vi "Receiver_Monokrom_Fix.vi"() -> ()   [LabVIEW 2018]
panel:
  in  "Python version":string="3.12.3"
  in  "Python Path Decoder Huffman":path=path "D:/PAKPRI_LAST/PAKPRI/huffman_decoder.py"
  out "Numeric":i32
  out "SNR":dbl
  out "Constellation Diagram Receiver":cdb[](graph)
  out "0, 2":i16[][](array[numeric])
  in  "Image File Reference":path=path "D:/Thesis Pak Pri/boo.bmp"
  out "x/y 3":dbl
  out "BER":dbl
  out "Output Image":picture
  in  "Width":i32=256
  in  "Height":i32=256
  out "Preamble Detected?":bool
  in  "Bit length (set)":i32=3600
  out "sisa bagi":i32
  out "hasil bagi":i32
  out "iterasi":i32
  in  "Modulation parameter":T1
  out "created new?":bool
  out "SIG valid?":bool
  in  "stop":bool
  out "USRP CoercedParamters":T2={"coerced IQ rate"=100000.0, "coerced carrier frequency"=100000.0, "coerced gain"=0.0} {"coerced gain" format="%#_6f"; "coerced carrier frequency" format="%#_6p"; "coerced IQ rate" format="%#_6p"}
  out "error out":errorcluster
  in  "Trigger level":dbl=0.005 format="%f"
  in  "error in (no error)":errorcluster
  in  "USRP ControledParameters":T3={"active antenna"="RX1", "gain"=0.0, "carrier frequency"=915000000.0, "IQ rate"=1000000.0} {"IQ rate" format="%#_6p"; "carrier frequency" format="%#_6p"; "gain" format="%#_6f"}
  in  "device names":refnum<k15>="192.168.10.4"
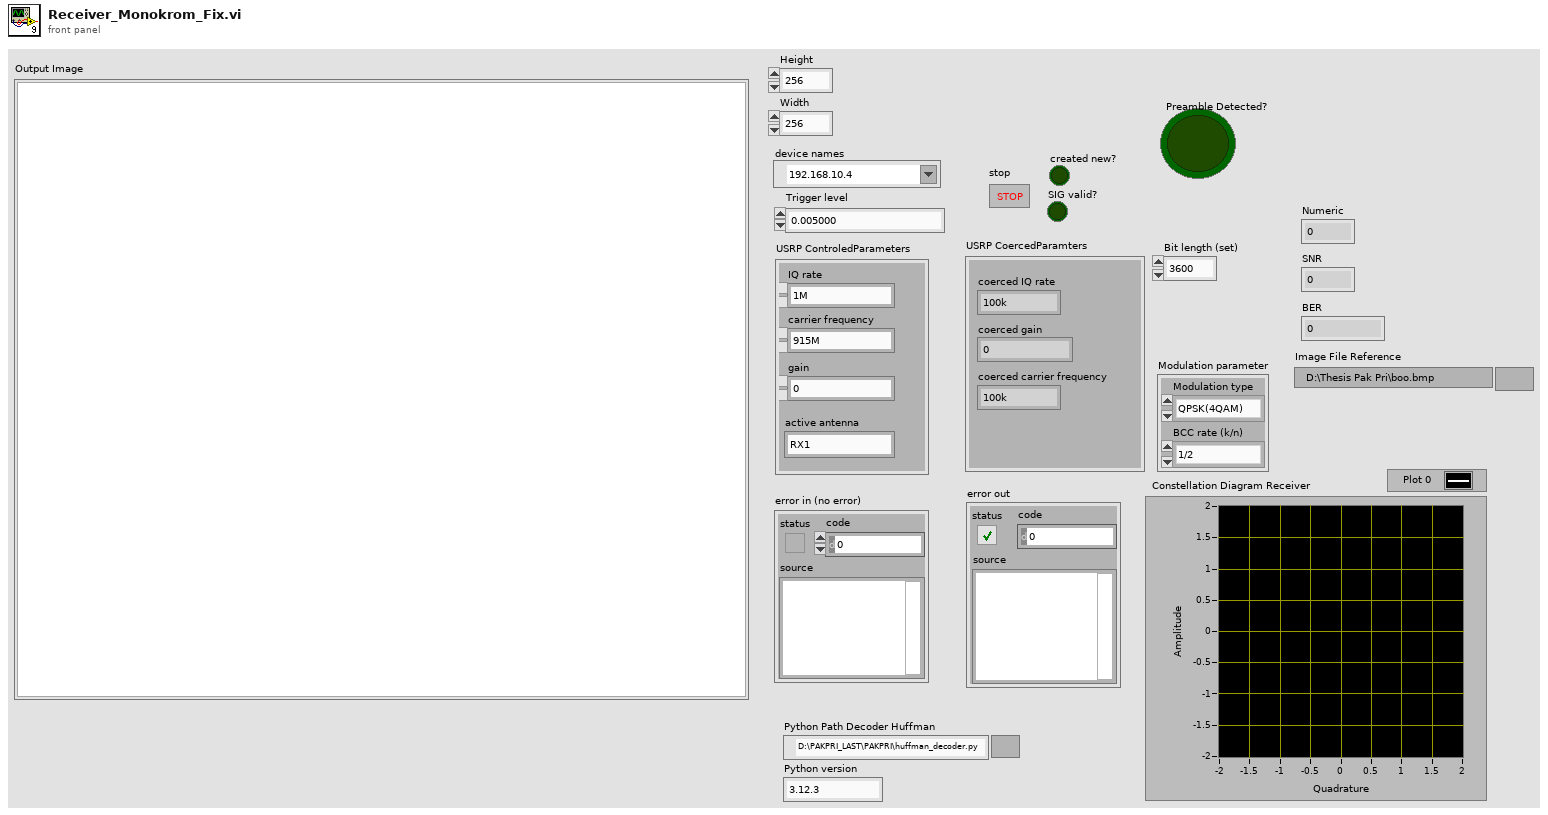
[diagram p1: front panel]
types:
  T1 = cluster{"Modulation type":enum16{"QPSK(4QAM)", "64QAM", "16QAM", "BPSK"}, "BCC rate (k/n)":enum16{"1/2", "2/3", "3/4"}}
  T2 = cluster{"coerced IQ rate":dbl, "coerced carrier frequency":dbl, "coerced gain":dbl}
  T3 = cluster{"active antenna":string, "gain":dbl, "carrier frequency":dbl, "IQ rate":dbl}
  T4 = typedef "imagedata.ctl" = cluster{"image type":i32, "image depth":i32, "image":u8[], "mask":u8[], "colors":u32[], "Rectangle":cluster{"left":i16, "top":i16, "right":i16, "bottom":i16}}
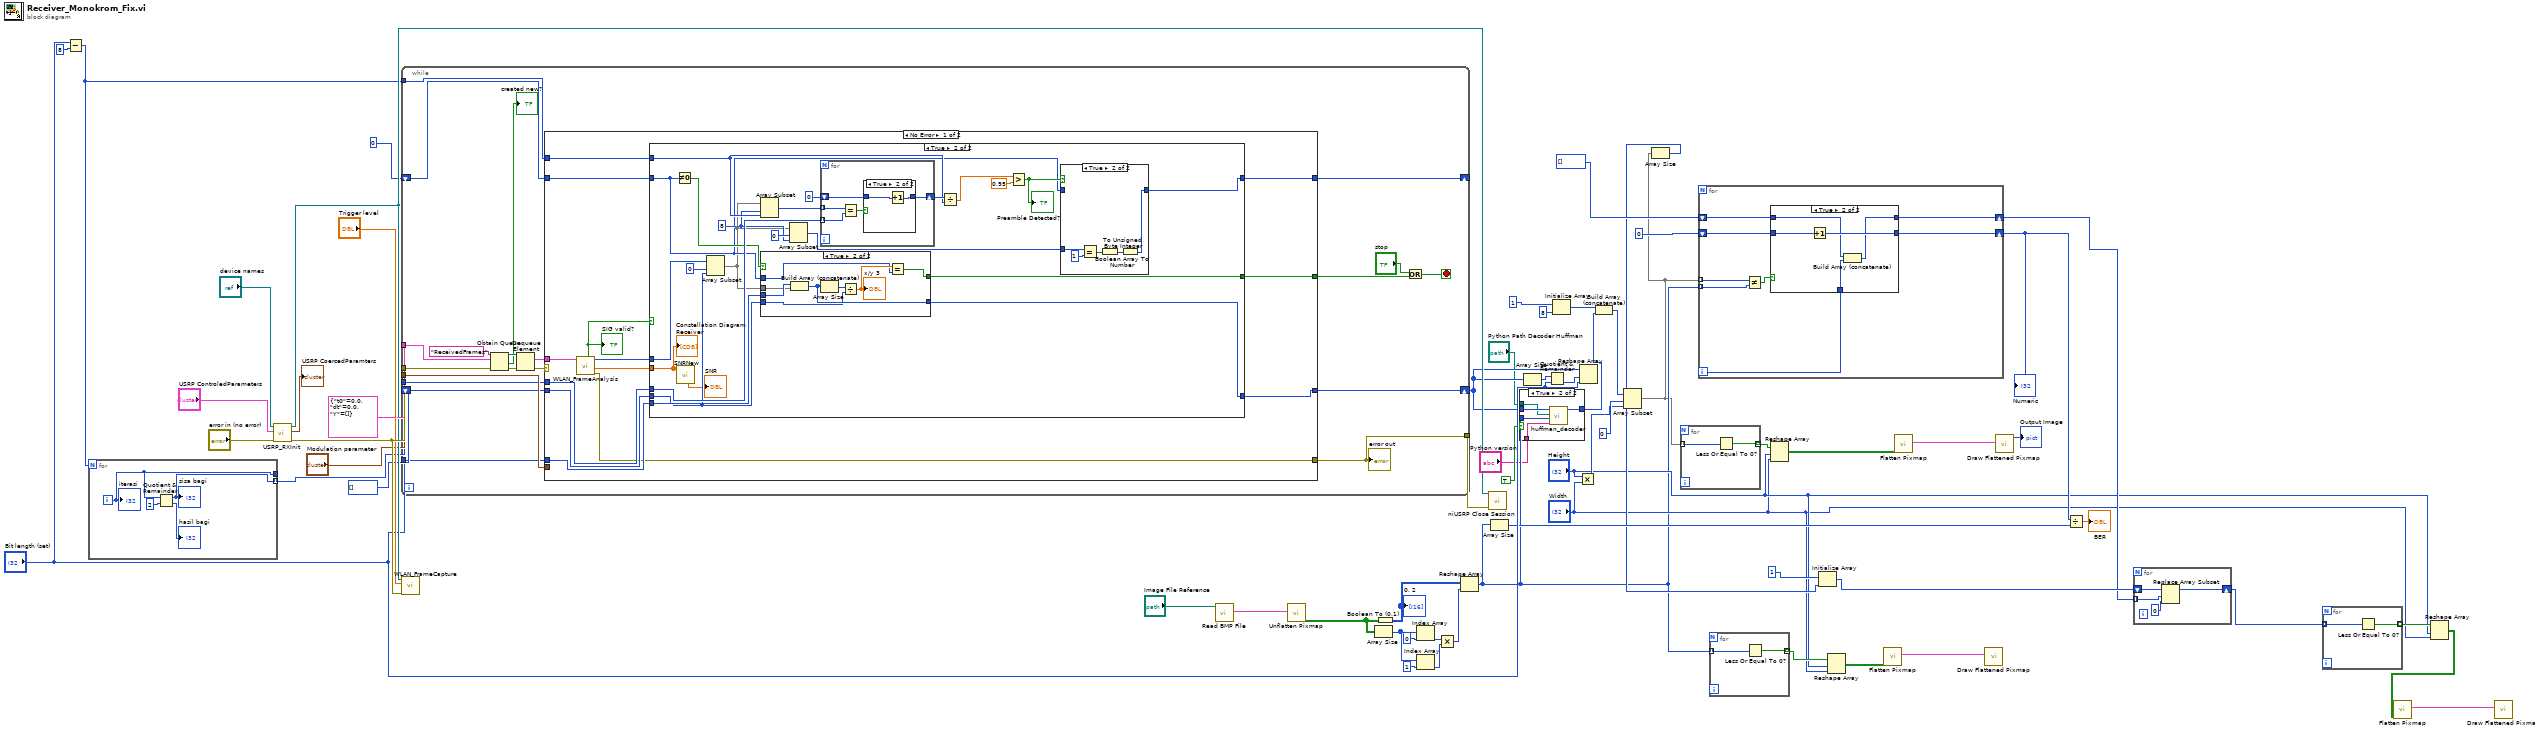
[diagram p0: block diagram]
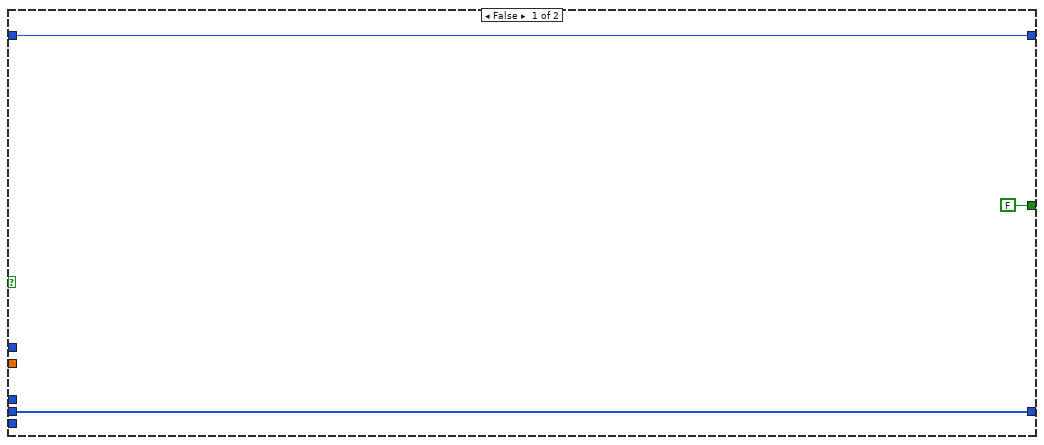
[diagram p4: hidden frame]
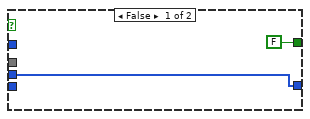
[diagram p5: hidden frame]
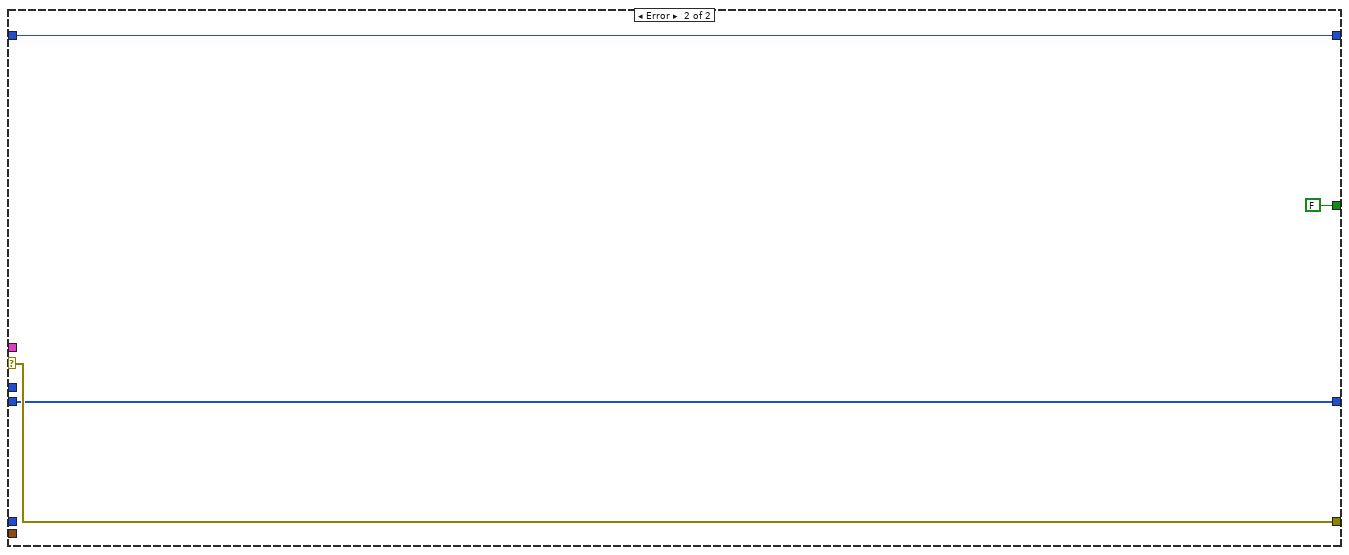
[diagram p8: hidden frame]
diagram:
  n1 = Subtract(x="Bit length (set)", y=8) -> (x-y=w52:i32)
  n2 = for {
    N: w52 -> [_]
    tunnel: [w65] -> _
    tunnel: [w64] -> w51 mode=indexing
    i -> [w65]
    n3 = Quotient & Remainder(x=w65, y=2) -> (x-y*floor(x/y)=w64:i32, floor(x/y)=→"hasil bagi":i32)
    "sisa bagi" <- w64
    "iterasi" <- w65
  }
  n4 = call "USRP_RXInit.vi"("device names"="device names", "USRP ControledParameters"="USRP ControledParameters", "error in (no error)"="error in (no error)") -> ("session handle out"=w55:refnum<k15>, "USRP CoercedParamters"=→"USRP CoercedParamters":T2, "error out"=w59:errorcluster)  [unwired: 5 in]
  n5 = while {
    tunnel: w59 -> [w86]
    tunnel: cluster{"t0":dbl, "dt":dbl, "Y":cdb[]} {"t0"=0.0, "dt"=0.0, "Y"=[]} ("data") -> [w87]
    tunnel: [w79] -> w56
    tunnel: "Modulation parameter" -> [w78]
    tunnel: "Bit length (set)" -> [w77]
    tunnel: w52 -> [w76]
    tunnel: w51 -> [w75]
    shift-right: [w73] -> _
    shift-left: 0 -> [w74]
    shift-right: [w71] -> w25
    shift-left: i32[] [] -> [w72]
    stop <- w68 stop-if-true
    n6 = Obtain Queue(name (unnamed)="ReceivedFrames", element data type=w87, error in (no error)=w86) -> (queue out=w85:refnum<queue>, created new?=→"created new?":bool, error out=w82:errorcluster)  [unwired: 2 in]
    n7 = Dequeue Element(queue=w85, error in (no error)=w82) -> (element=w83:cluster{"t0":dbl, "dt":dbl, "Y":cdb[]}, error out=w84:errorcluster)  [unwired: 1 in, 2 out]
    n8 = case shown="No Error" w84 {
      selector: w84 -> [_ w154]
      tunnel: w83 -> [w92 _]
      tunnel: [w91 w154] -> w79
      tunnel: w78 -> [_ _]
      tunnel: w77 -> [w100 _]
      tunnel: w76 -> [w99 _]
      tunnel: w75 -> [w98 _]
      tunnel: w74 -> [w97 w153]
      tunnel: [w96 w153] -> w73
      tunnel: w72 -> [w95 w152]
      tunnel: [w94 w152] -> w71
      tunnel: [w93 FALSE] -> w69
      frame No Error {
        n9 = call "WLAN_FrameAnalysis.vi"("input cluster"=w92) -> ("error out"=w91:errorcluster, "Constellation"=w88:cdb[], "output bits"=w89:i8[], "SIG valid?"=w90:bool)  [unwired: 5 in, 2 out]
        "SIG valid?" <- w90
        n10 = case shown="True" w90 {
          tunnel: w89 -> [_ w106]
          tunnel: w88 -> [_ w105]
          tunnel: w100 -> [_ w112]
          tunnel: w99 -> [_ w121]
          tunnel: w98 -> [_ w124]
          tunnel: w97 -> [w103 w111]
          tunnel: [w103 w115] -> w96
          tunnel: w95 -> [w102 w113]
          tunnel: [w102 w109] -> w94
          tunnel: [FALSE w110] -> w93
          frame False {
          }
          frame True {
            w117 = 8 ("index")
            n11 = Not Equal To 0?(x=w111) -> (x != 0?=w114:bool)
            n12 = call "SNRNew.vi"("Constellation"=w105) -> ("SNR"=→"SNR":dbl)  [unwired: 7 in, 3 out]
            n13 = Array Subset(array=w106, index=0, length=w112) -> (w107:i8[])
            n14 = Array Subset(array=w107, index=w117, length=w121) -> (w125:i8[])
            n15 = case shown="True" w114 {
              tunnel: w113 -> [w128 w136]
              tunnel: w107 -> [_ w135]
              tunnel: [w128 w132] -> w109
              tunnel: w112 -> [_ w131]
              tunnel: w111 -> [_ w130]
              tunnel: [FALSE w129] -> w110
              frame False {
              }
              frame True {
                n16 = Build Array (concatenate)(w136, w135) -> (w132:i32[])
                n17 = Array Size(array=w132) -> (size(s)=w134:i32)
                n18 = Divide(x=w134, y=w131) -> (x/y=w133:dbl)
                "x/y 3" <- w133
                n19 = Equal?(x=w133, y=w130) -> (x = y?=w129:bool)
              }
            }
            n20 = Array Subset(array=w107, index=0, length=w117) -> (w116:i8[])
            n21 = for {
              tunnel: w125 -> [w146] mode=indexing
              tunnel: w124 -> [w147] mode=indexing
              shift-right: [w143] -> w122
              shift-left: 0 -> [w144]
              n22 = Equal?(x=w146, y=w147) -> (x = y?=w145:bool)
              n23 = case shown="True" w145 {
                tunnel: w144 -> [w148 w150]
                tunnel: [w148 w149] -> w143
                frame False {
                }
                frame True {
                  n24 = Increment(x=w150) -> (x+1=w149:i32)
                }
              }
            }
            n25 = Divide(x=w122, y=w121) -> (x/y=w108:dbl)
            n26 = Greater?(x=w108, y=0.95) -> (0:w119:bool)
            "Preamble Detected?" <- w119
            n27 = case shown="True" w119 {
              tunnel: w116 -> [_ w140]
              tunnel: w111 -> [w137 _]
              tunnel: [w137 w138] -> w115
              frame False {
              }
              frame True {
                n28 = Equal?(x=w140, y=1) -> (x = y?=w141:bool[])
                n29 = Boolean Array To Number(Boolean array=w141) -> (number=w139:u32)
                n30 = To Unsigned Byte Integer(number=w139) -> (unsigned 8bit integer=w138:u8)
              }
            }
            "Constellation Diagram Receiver" <- w105
          }
        }
      }
      frame Error {
      }
    }
    "error out" <- w79
    n31 = Or(x="stop", y=w69) -> (x .or. y?=w68:bool)
  }
  n32 = call "WLAN_FrameCapture.vi"("error in (no error)"=w59, "Trigger level"="Trigger level", "session handle"=w55) -> ()  [unwired: 8 in]
  n33 = call <vilib>:"Read BMP File.vi"("path to BMP file"="Image File Reference") -> ("image data"=w34:T4)  [unwired: 8 in, 2 out]
  n34 = call <vilib>:"Unflatten Pixmap.vi"("image data"=w34) -> ("1-bit pixmap"=w32:bool[][])  [unwired: 4 in, 6 out]
  n35 = Array Size(array=w32) -> (size(s)=w29:i32[])
  n36 = Boolean To (0,1)(Boolean=w32) -> (0, 1=w33:i16[][])
  "0, 2" <- w33
  n37 = Index Array(array=w29, index=0) -> (element=w28:i32)
  n38 = Index Array(array=w29, index=1) -> (element=w27:i32)
  n39 = Multiply(x=w28, y=w27) -> (x*y=w26:i32)
  n40 = Reshape Array(w33, w26) -> (w9:i16[])
  n41 = call <instrlib>:"niUSRP Close Session.vi"("session handle"=w55, "error in (no error)"=w56) -> ()  [unwired: 13 in, 1 out]
  n42 = Array Size(array=w9) -> (size(s)=w38:i32)
  n43 = case shown="True" TRUE {
    tunnel: w25 -> [w155 w160]
    tunnel: [w155 w159] -> w4
    tunnel: w9 -> [_ w158]
    tunnel: "Python Path Decoder Huffman" -> [_ w157]
    tunnel: "Python version" -> [_ w156]
    frame False {
    }
    frame True {
      n44 = call "huffman_decoder.vi"("Python version"=w156, "data_array_bit"=w158, "module path"=w157, "encode_array_bit"=w160) -> ("return value"=w159:i32[])  [unwired: 7 in]
    }
  }
  n45 = Array Size(array=w25) -> (size(s)=w48:i32)
  n46 = Quotient & Remainder(x=w48, y="Bit length (set)") -> (floor(x/y)=w42:i32)  [unwired: 1 out]
  n47 = Initialize Array(1, 8 ("dimension size")) -> (w5:i32[])
  n48 = Multiply(x="Height", y="Width") -> (x*y=w43:i32)
  n49 = Reshape Array(w25, w42, "Bit length (set)") -> ()  [unwired: 1 out]
  n50 = Build Array (concatenate)(w5, w4) -> (w3:i32[])
  n51 = Array Subset(array=w3, index=0, length=w43) -> (w8:i32[])
  n52 = Array Size(array=w8) -> (size(s)=w21:i32)
  n53 = for {
    tunnel: w8 -> [w162] mode=indexing
    tunnel: [w161] -> w46 mode=indexing
    n54 = Less Or Equal To 0?(x=w162) -> (x <= 0?=w161:bool)
  }
  n55 = for {
    tunnel: w8 -> [w170] mode=indexing
    tunnel: w9 -> [w169] mode=indexing
    shift-right: [w166] -> w39
    shift-left: 0 -> [w167]
    shift-right: [w163] -> w19
    shift-left: i32[] [] -> [w165]
    i -> [w164]
    n56 = Not Equal?(x=w170, y=w169) -> (x != y?=w168:bool)
    n57 = case shown="True" w168 {
      tunnel: w167 -> [w172 w177]
      tunnel: [w172 w176] -> w166
      tunnel: w165 -> [w171 w175]
      tunnel: w164 -> [_ w174]
      tunnel: [w171 w173] -> w163
      frame False {
      }
      frame True {
        n58 = Increment(x=w177) -> (x+1=w176:i32)
        n59 = Build Array (concatenate)(w175, w174) -> (w173:i32[])
      }
    }
  }
  "Numeric" <- w39
  n60 = for {
    tunnel: w9 -> [w179] mode=indexing
    tunnel: [w178] -> w14 mode=indexing
    n61 = Less Or Equal To 0?(x=w179) -> (x <= 0?=w178:bool)
  }
  n62 = Reshape Array(w46, "Height", "Width") -> (w45:bool[][])
  n63 = Initialize Array(1, w21) -> (w20:i32[])
  n64 = Reshape Array(w14, "Height", "Width") -> (w10:bool[][])
  n65 = call <vilib>:"Flatten Pixmap.vi"("1-bit pixmap"=w10) -> ("image data"=w11:T4)  [unwired: 10 in]
  n66 = call <vilib>:"Flatten Pixmap.vi"("1-bit pixmap"=w45) -> ("image data"=w47:T4)  [unwired: 10 in]
  n67 = call <vilib>:"Draw Flattened Pixmap.vi"("image data"=w11) -> ()  [unwired: 8 in, 1 out]
  n68 = call <vilib>:"Draw Flattened Pixmap.vi"("image data"=w47) -> ("new picture"=→"Output Image":picture)  [unwired: 8 in]
  n69 = Divide(x=w39, y=w38) -> (x/y=→"BER":dbl)
  n70 = for {
    tunnel: w19 -> [w182] mode=indexing
    shift-right: [w180] -> w18
    shift-left: w20 -> [w183]
    n71 = Replace Array Subset(array=w183, new element=0 ("new element/subarray"), index=w182) -> (w180:i32[])
  }
  n72 = for {
    tunnel: w18 -> [w185] mode=indexing
    tunnel: [w184] -> w17 mode=indexing
    n73 = Less Or Equal To 0?(x=w185) -> (x <= 0?=w184:bool)
  }
  n74 = Reshape Array(w17, "Height", "Width") -> (w15:bool[][])
  n75 = call <vilib>:"Flatten Pixmap.vi"("1-bit pixmap"=w15) -> ("image data"=w16:T4)  [unwired: 10 in]
  n76 = call <vilib>:"Draw Flattened Pixmap.vi"("image data"=w16) -> ()  [unwired: 8 in, 1 out]
